vi "LIA Sideband Noise.vi"(9 "length":i32, 10 "index":i32, 11 "Power Spectrum / PSD (dBm) in":cluster{"f0":dbl, "df":dbl, "magnitude":dbl[]}) -> (2 "Numeric Control":dbl, 3 "Power Spectrum / PSD (dBm) out":cluster{"f0":dbl, "df":dbl, "magnitude":dbl[]})   [LabVIEW 2018]
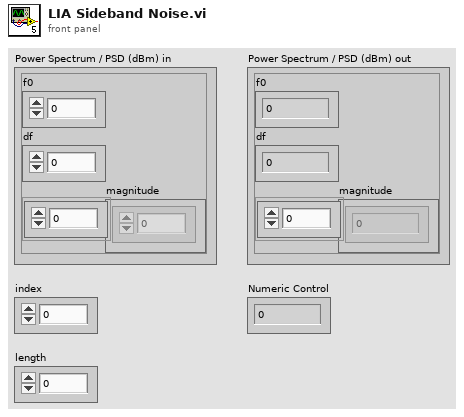
[diagram p1: front panel]
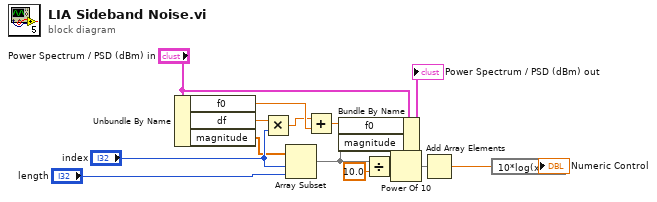
[diagram p0: block diagram]
diagram:
  n1 = Unbundle By Name("Power Spectrum / PSD (dBm) in") -> ("f0"=w8:dbl, "df"=w5:dbl, "magnitude"=w2:dbl[])
  n2 = Multiply(x=w5, y="index") -> (x*y=w6:dbl)
  n3 = Array Subset(array=w2, index="index", length="length") -> (w12:dbl[])
  n4 = Add(x=w6, y=w8) -> (x+y=w7:dbl)
  n5 = Bundle By Name(cluster="Power Spectrum / PSD (dBm) in", "f0"=w7, "magnitude"=w12) -> (→"Power Spectrum / PSD (dBm) out":cluster{"f0":dbl, "df":dbl, "magnitude":dbl[]})
  n6 = Divide(x=w12, y=10.0) -> (x/y=w10:dbl[])
  n7 = Power Of 10(x=w10) -> (10^x=w13:dbl[])
  n8 = Add Array Elements(numeric array=w13) -> (sum=w15:dbl)
  n9 = expression code="10*log(x)"(w15) -> (→"Numeric Control":dbl)
